vi "Fan Semaphore.vi"() -> (0 "Ring":u16(ring))   [LabVIEW 8.6]
doc: "Fan control demonstration (low res fan)\n\n(c) Copyright SGCTek 2003,2004 All rights reserved\nsgctek@hotmail.com\nhttp://members.lycos.co.uk/sgctek/\n\nPlease DO NOT distribute this control!!!\nBy, for example P2P, email, FTP, WEB or other techniques.\nPlease direct people to http://members.lycos.co.uk/sgctek/\n\nIf you use this software or control you must include a\ncopyright notice in your software and documentation \nincluding a statement indicating: -\n 'Portions (c) Copyright SGCTek 2003,2004 \n http://members.lycos.co.uk/sgctek/'\n\nProvided that you include the above notice you may distribute\nthis control or code as part of an Labview EXE or project.\n\n\nThis software is supplied on an 'AS IS' basis. No liabilty\nis accepted for errors or omissions. No responsability is\naccepted for loss or damage how so ever arising, consequential\nor otherwise. \n\nNo part of these systems may be used in conjunction with\nequipment associated with life support or where life may\nbe put at risk or possible injury occur as a result of error\nor failure in these modules / software or as a result of its\nuse. For example but not limited to medical applications,\nemergency stop systems or safety critical applications. \n\nDetermination as to fitness or suitability for purpose is\nentirely your responsability.\n\nAll registered trademarks are recognised as owned by thier\nrespective registrants."
panel:
  in  "FANSpeed":u32(slide)
  in  "2DArraySize":i32
  out "MainLoop":i32
  out "Array":i32[][](array[numeric])
  in  "Direction":bool
  in  "Exit":bool
  # "fast"
  # "slow"
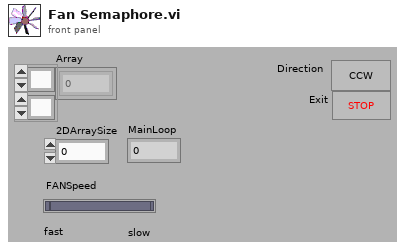
[diagram p1: front panel]
types:
  T1 = typedef "Semaphore RefNum" = refnum<k1>
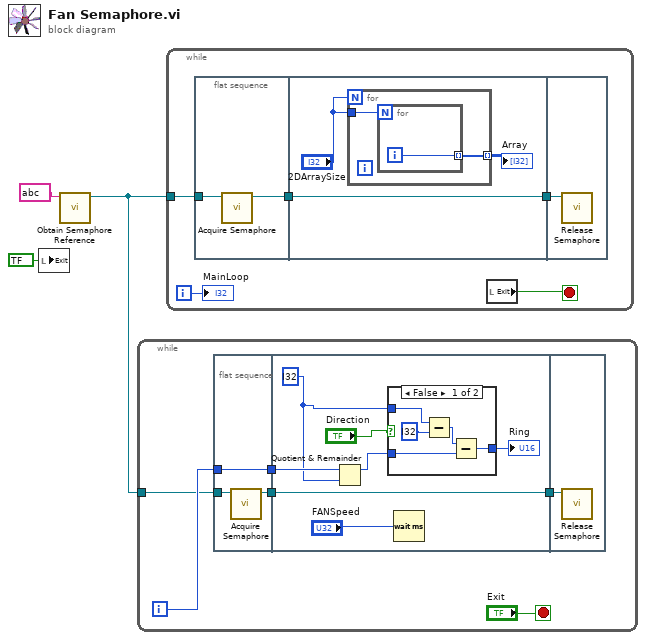
[diagram p0: block diagram]
diagram:
  n1 = local write "Exit"(bool ? ("Exit")) -> ()
  n2 = call <vilib>:"Obtain Semaphore Reference.vi"("name (unnamed)"=string ?) -> ("semaphore"=w2:T1)  [unwired: 4 in, 2 out]
  n3 = while {
    tunnel: w2 -> [w6]
    i -> [w8]
    stop <- "Exit" stop-if-true
    n4 = flat-sequence {
      tunnel: w8 -> [w12]
      tunnel: [w12] -> w7
      tunnel: w6 -> [w11]
      tunnel: [w10] -> w4
      tunnel: w7 -> [w17]
      tunnel: [w14] -> w5
      tunnel: w4 -> [w14]
      tunnel: w5 -> [w26]
      frame #0 {
        n5 = call <vilib>:"Acquire Semaphore.vi"("semaphore"=w11) -> ("semaphore out"=w10:T1)  [unwired: 4 in, 2 out]
      }
      frame #1 {
        w16 = i32 ?
        n6 = Quotient & Remainder(x=w17, y=w16) -> (x-y*floor(x/y)=w15:i32)  [unwired: 1 out]
        n7 = case shown="False" "Direction" {
          tunnel: [w24 w25] -> w19
          tunnel: w15 -> [w23 w25]
          tunnel: w16 -> [w21 _]
          frame #0 {
            n8 = Subtract(x=w21, y=i32 ?) -> (x-y=w22:i32)
            n9 = Subtract(x=w22, y=w23) -> (x-y=w24:i32)
          }
          frame #1 {
          }
        }
        "Ring" <- w19
        n10 = Wait (ms)(milliseconds to wait="FANSpeed") -> ()  [unwired: 1 out]
      }
      frame #2 {
        n11 = call <vilib>:"Release Semaphore.vi"("semaphore"=w26) -> ()  [unwired: 5 in, 2 out]
      }
    }
  }
  n12 = while {
    tunnel: w2 -> [w29]
    i -> [w30]
    stop <- w31 stop-if-true
    n13 = flat-sequence {
      tunnel: w29 -> [w33]
      tunnel: [w32] -> w28
      tunnel: w28 -> [w34]
      tunnel: [w34] -> w27
      tunnel: w27 -> [w40]
      frame #0 {
        n14 = call <vilib>:"Acquire Semaphore.vi"("semaphore"=w33) -> ("semaphore out"=w32:T1)  [unwired: 4 in, 2 out]
      }
      frame #1 {
        n15 = for {
          N: "2DArraySize" -> [_]
          tunnel: "2DArraySize" -> [w38]
          tunnel: [w37] -> w35 mode=indexing
          n16 = for {
            N: w38 -> [_]
            tunnel: [w39] -> w37 mode=indexing
            i -> [w39]
          }
        }
        "Array" <- w35
      }
      frame #2 {
        n17 = call <vilib>:"Release Semaphore.vi"("semaphore"=w40) -> ()  [unwired: 5 in, 2 out]
      }
    }
    n18 = local read "Exit"() -> (w31:bool)
    "MainLoop" <- w30
  }
